vi "Inlet Convert Temp to Volt HAWK.vi"(1 "Inlet Temperature":dbl) -> (0 "Inlet Voltage":dbl)   [LabVIEW 2014]
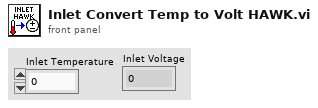
[diagram p1: front panel]
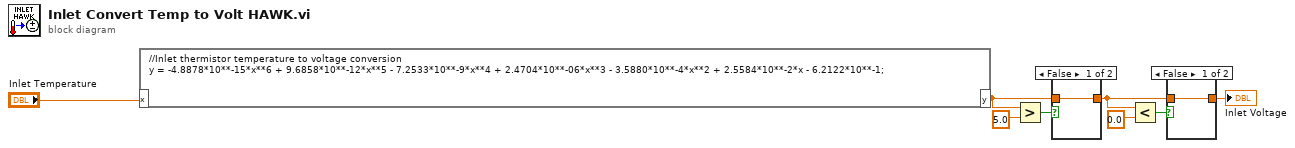
[diagram p0: block diagram]
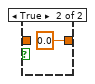
[diagram p2: hidden frame]
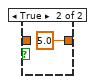
[diagram p3: hidden frame]
diagram:
  n1 = formula code="//Inlet thermistor temperature to voltage conversion\ny = -4.8878*10**-15*x**6 + 9.6858*10**-12*x**5 - 7.2533*10**-9*x**4 + 2.4704*10**-06*x**3 - 3.5880*10**-4*x**2 + 2.5584*10**-2*x - 6.2122*10**-1;"("x"="Inlet Temperature") -> ("y"=w5:dbl)
  n2 = Greater?(x=w5, y=5.0) -> (0:w3:bool)
  n3 = case shown="False" w3 {
    tunnel: [w9 5.0 ("y")] -> w8
    tunnel: w5 -> [w9 _]
    frame False {
    }
    frame True {
    }
  }
  n4 = Less?(x=w8, y=0.0) -> (x < y?=w7:bool)
  n5 = case shown="False" w7 {
    tunnel: [w11 0.0 ("y")] -> w1
    tunnel: w8 -> [w11 _]
    frame False {
    }
    frame True {
    }
  }
  "Inlet Voltage" <- w1
